vi "FUG-HCN.SetOnOff.vi"(0 "i ref in":refnum<vi>, 2 "Time out":i32, 3 "on (FALSE)":bool, 5 "error in (no error)":errorcluster) -> (14 "i ref out":refnum<vi>, 19 "error out":errorcluster)   [LabVIEW 2014, in "FUG-HCN.lvlib"]
doc: "Enables or disables remote control."
uses:
  FUG-HCN.lvlib
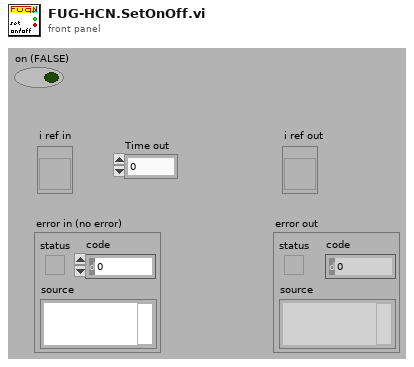
[diagram p1: front panel]
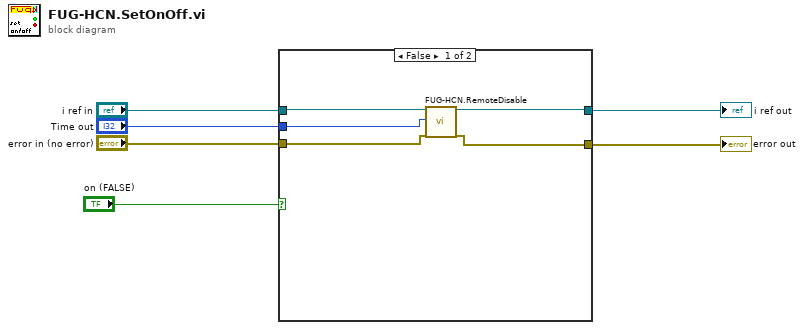
[diagram p0: block diagram]
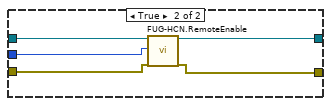
[diagram p2: hidden frame]
diagram:
  n1 = case shown="False" "on (FALSE)" {
    tunnel: "i ref in" -> [w11 w16]
    tunnel: [w10 w15] -> w4
    tunnel: [w9 w14] -> w3
    tunnel: "error in (no error)" -> [w8 w13]
    tunnel: "Time out" -> [w7 w12]
    frame False {
      n2 = call "FUG-HCN.RemoteDisable.vi"("i ref in"=w11, "Time out"=w7, "error in (no error)"=w8) -> ("i ref out"=w10:refnum<vi>, "error out"=w9:errorcluster)  [unwired: 14 in, 1 out]
    }
    frame True {
      n3 = call "FUG-HCN.RemoteEnable.vi"("i ref in"=w16, "Time out"=w12, "error in (no error)"=w13) -> ("i ref out"=w15:refnum<vi>, "error out"=w14:errorcluster)  [unwired: 14 in, 1 out]
    }
  }
  "error out" <- w3
  "i ref out" <- w4
